vi "cRIO Test ftp webDAV installed.vi"() -> (1 "WebDAV":bool, 3 "ftp":bool)   [LabVIEW 2020, in "Backup.lvlib"]
uses:
  Backup.lvlib
  <vilib>/nisyscfg/Get Installed Components.vi
  <vilib>/nisyscfg/Close (System).vi
  <vilib>/nisyscfg/nisyscfg.lvlib
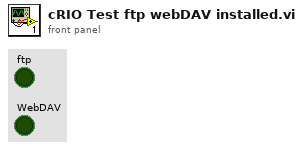
[diagram p1: front panel]
types:
  T1 = typedef "nisyscfg.lvlib/Software 1.2.ctl" = cluster{"title":string, "description":string, "ID":string, "version":string, "component type":T2}
  T2 = typedef "nisyscfg.lvlib/Component Type.ctl" = u32
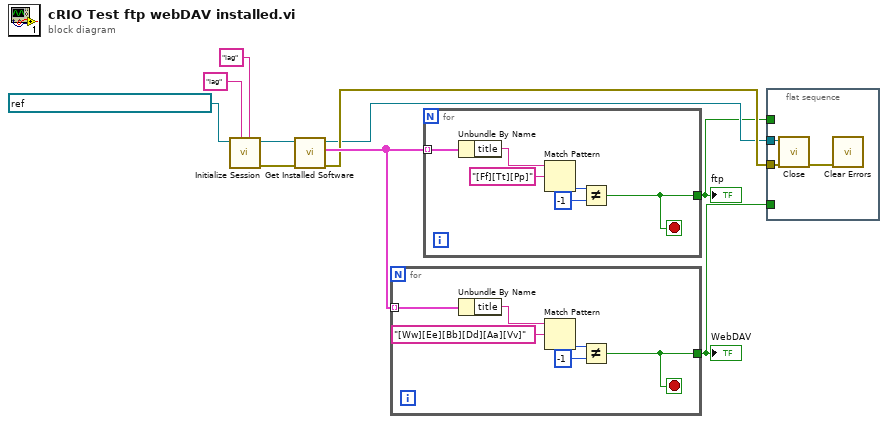
[diagram p0: block diagram]
diagram:
  n1 = call <vilib>:"Initialize Session.vi"("Password"="iag", "User Name"="iag", "Target (localhost)"=refnum<k21> "NI-cRIO-9066-IAG (192.168.14.14)") -> ("error out"=w6:errorcluster, "Session out"=w7:refnum<k21>)  [unwired: 7 in]
  n2 = call-poly <vilib>:"Get Installed Software.vi"("error in (no error)"=w6, "Session in"=w7) -> ("error out"=w4:errorcluster, "Software Components"=w5:T1[], "Session out"=w3:refnum<k21>)  [unwired: 7 in]
  n3 = for {
    tunnel: w5 -> [w16] mode=indexing
    tunnel: [w11] -> w1
    stop <- w11 stop-if-true
    n4 = Unbundle By Name(w16) -> ("title"=w15:string)
    n5 = Match Pattern(string=w15, regular expression="[Ww][Ee][Bb][Dd][Aa][Vv]" ("Regulärer Ausdruck")) -> (offset past match=w13:i32)  [unwired: 1 in, 3 out]
    n6 = Not Equal?(x=w13, y=-1) -> (x != y?=w11:bool)
  }
  "WebDAV" <- w1
  n7 = for {
    tunnel: w5 -> [w22] mode=indexing
    tunnel: [w17] -> w2
    stop <- w17 stop-if-true
    n8 = Unbundle By Name(w22) -> ("title"=w21:string)
    n9 = Match Pattern(string=w21, regular expression="[Ff][Tt][Pp]" ("Regulärer Ausdruck")) -> (offset past match=w19:i32)  [unwired: 1 in, 3 out]
    n10 = Not Equal?(x=w19, y=-1) -> (x != y?=w17:bool)
  }
  "ftp" <- w2
  n11 = flat-sequence {
    tunnel: w4 -> [w25]
    tunnel: w3 -> [w24]
    tunnel: w2 -> [_]
    tunnel: w1 -> [_]
    frame #0 {
      n12 = call-poly <vilib>:"Close.vi"("error in (no error)"=w25, "Session in"=w24) -> ("error out"=w23:errorcluster)  [unwired: 9 in]
      n13 = call <vilib>:"Clear Errors.vi"("error in (no error)"=w23) -> ()  [unwired: 5 in, 2 out]
    }
  }
